vi "Open Hardware.vi"(8 "error in (no error)":errorcluster, 11 "Inst.Magneto in":refnum<class "Inst.Magneto.lvclass">) -> (0 "error out":errorcluster, 3 "Inst.Magneto out":refnum<class "Inst.Magneto.lvclass">)   [LabVIEW 2019, in "Inst.Magneto.lvclass"]
uses:
  Inst.Magneto.lvclass
  <userlib>/LevyLab/Instrument Framework/Instrument Types/VSource/Instrument.VSource.lvclass
  <vilib>/httpClient/LabVIEWHTTPClient.lvlib
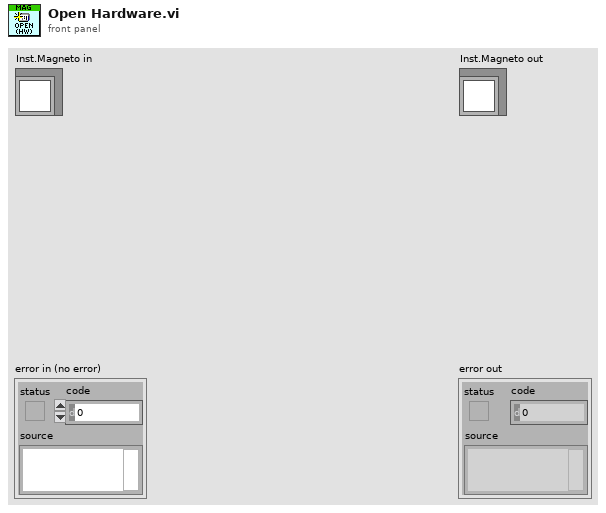
[diagram p1: front panel]
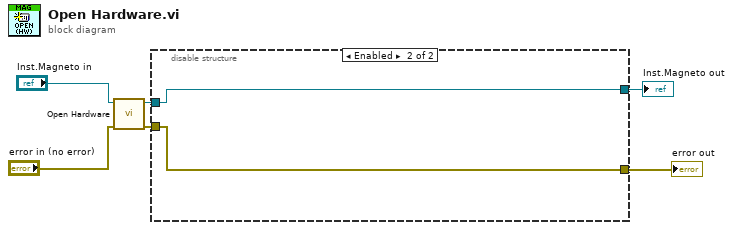
[diagram p0: block diagram]
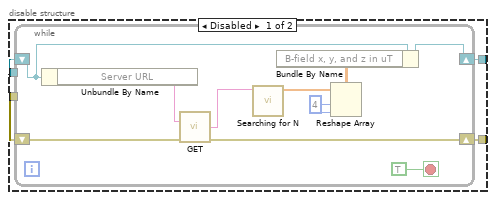
[diagram p2: hidden frame]
diagram:
  n1 = call-parent "Open Hardware.vi"("error in (no error)"="error in (no error)", "Instrument in"="Inst.Magneto in") -> ("error out"=w2:errorcluster, "Instrument out"=w4:refnum<class "Inst.Magneto.lvclass">)  [unwired: 8 in]
  n2 = disable-structure shown="Enabled" {
    disable-tunnel: [w10 w21] -> w5
    disable-tunnel: w4 -> [w9 w22]
    disable-tunnel: w2 -> [w8 w21]
    disable-tunnel: [w7 w22] -> w1
    frame Disabled {
      n3 = while {
        shift-right: [w18] -> w7
        shift-left: w9 -> [w12]
        shift-right: [w19] -> w10
        shift-left: w8 -> [w13]
        stop <- TRUE stop-if-true
        w16 = 4 ("dimension size")
        n4 = Unbundle By Name(w12) -> ("Server URL"=w20:string)
        n5 = call <vilib>:"GET.vi"("url"=w20, "error in (no error)"=w13) -> ("body"=w17:string, "error out"=w19:errorcluster)  [unwired: 10 in, 2 out]
        n6 = call "Searching for N.vi"("body"=w17) -> ("Array"=w15:dbl[])  [unwired: 10 in]
        n7 = Reshape Array(w15, w16, w16) -> (w14:dbl[][])
        n8 = Bundle By Name(cluster=w12, "B-field x, y, and z in uT"=w14) -> (w18:refnum<class "Inst.Magneto.lvclass">)
      }
    }
    frame Enabled {
    }
  }
  "error out" <- w5
  "Inst.Magneto out" <- w1
